vi "new_success.vi"(8 "error out":errorcluster) -> (3 "result":T1)   [LabVIEW 2015]
uses:
  tester_result.ctl
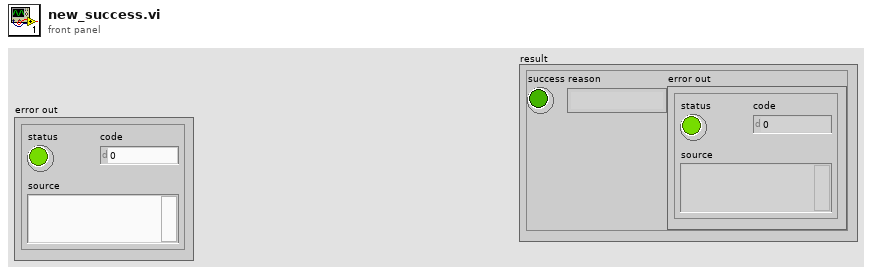
[diagram p1: front panel]
types:
  T1 = typedef "tester_result.ctl" = cluster{"success":bool, "reason":string, "error out":errorcluster}
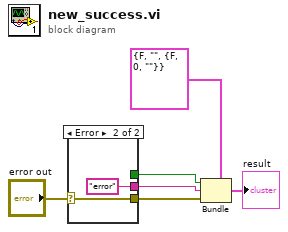
[diagram p0: block diagram]
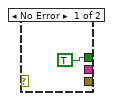
[diagram p2: hidden frame]
diagram:
  n1 = case shown="Error" "error out" {
    selector: "error out" -> [_ w9]
    tunnel: [_ w9] -> w3
    tunnel: [TRUE _] -> w2
    tunnel: [_ "error" ("reason")] -> w1
    frame No Error {
    }
    frame Error {
    }
  }
  n2 = Bundle(cluster=T1 {"success"=FALSE, "reason"="", "error out"={"status"=FALSE, "code"=0, "source"=""}} ("test_result"), "success"=w2, "reason"=w1, "error out"=w3) -> (→"result":T1)
